vi "EncryptionDecorator_Create.vi"(8 "error in (no error)":errorcluster, 10 "Source":refnum<class "DataSource.lvclass">, 11 "reference in":refnum<class "EncryptionDecorator.lvclass">) -> (0 "error out":errorcluster, 3 "reference out":refnum<class "EncryptionDecorator.lvclass">)   [LabVIEW 2020, in "EncryptionDecorator.lvclass"]
uses:
  EncryptionDecorator.lvclass
  C:/Projects/OpenGDS_DesignPatterns/Decorator3/DataSourceDecorator_class/DataSourceDecorator.lvclass
  DataSource_interface/DataSource.lvclass
  DataSourceDecorator_class/DataSourceDecorator.lvclass
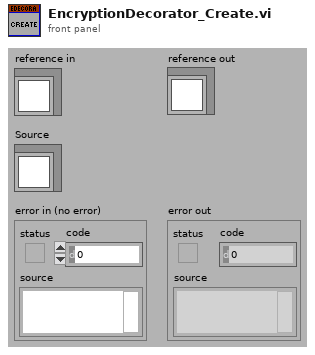
[diagram p1: front panel]
types:
  T1 = typedef "EncryptionDecorator.lvclass/ObjectAttributes.ctl" = cluster{"None":bool}
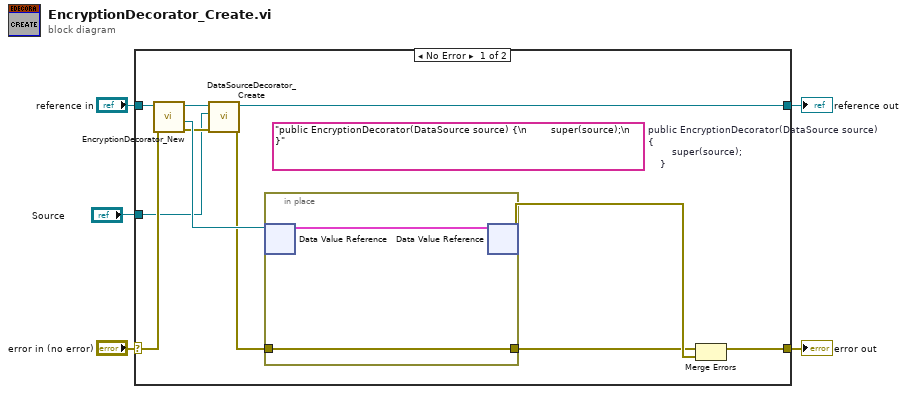
[diagram p0: block diagram]
diagram:
  n1 = case shown="No Error" "error in (no error)" {
    selector: "error in (no error)" -> [w12 w20]
    tunnel: [w10 w20] -> w4
    tunnel: "reference in" -> [w14 w19]
    tunnel: [w9 w19] -> w2
    tunnel: "Source" -> [w6 _]
    frame No Error {
      (unwired) "public EncryptionDecorator(DataSource source) {\n        super(source);\n    }"  # public EncryptionDecorator(DataSource source) {         super(source);     }
      n2 = call "EncryptionDecorator_New.vi"("error in (no error)"=w12, "reference in"=w14) -> ("error out"=w13:errorcluster, "DVRRefOut"=w16:refnum<data-value>, "reference out"=w15:refnum<class "EncryptionDecorator.lvclass">)  [unwired: 6 in, 1 out]
      n3 = call "DataSourceDecorator_Create.vi"("error in (no error)"=w13, "Source"=w6, "reference in"=w15) -> ("error out"=w8:errorcluster, "reference out"=w9:refnum<class "EncryptionDecorator.lvclass">)  [unwired: 7 in]
      n4 = in-place {
        in-place-border: w8 -> [w18]
        in-place-border: [w18] -> w7
        n5 = in-place-dvr #1(w16) -> (w17:T1)  [unwired: 1 out]
        n6 = in-place-dvr #1(w17) -> (w11:errorcluster)  [unwired: 1 out]
      }
      n7 = Merge Errors(w7, w11) -> (w10:errorcluster)
    }
    frame Error {
    }
  }
  "error out" <- w4
  "reference out" <- w2
